vi "SMTP Email Get Literal Search Pattern.vi"(2 "case matching (sensitive)":T1=enum."system", 3 "literal string":string) -> (1 "regular expression":string)   [LabVIEW 2011, in "NewNI_SMTPEmail.lvlib"]
doc: "Builds a regular expression (used by Match Pattern) to match a literal string.\n\nWhen match case is FALSE, the regular expression will perform a case-insensitive match."
uses:
  NewNI_SMTPEmail.lvlib
  SMTP Email Case Matching.ctl
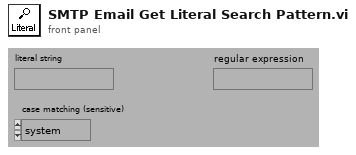
[diagram p1: front panel]
types:
  T1 = typedef "NewNI_SMTPEmail.lvlib/SMTP Email Case Matching.ctl" = enum16{"a != A", "a == A", "system"}
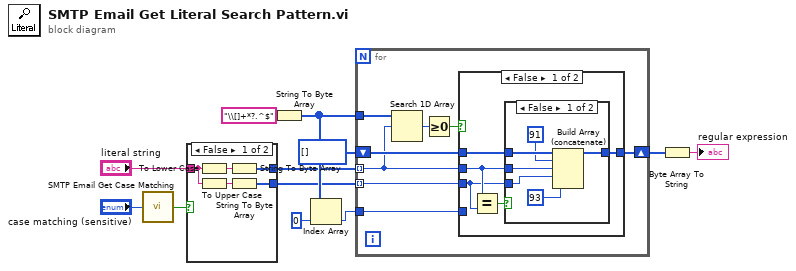
[diagram p0: block diagram]
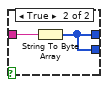
[diagram p2: hidden frame]
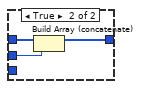
[diagram p3: hidden frame]
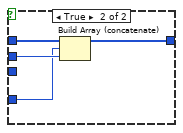
[diagram p4: hidden frame]
diagram:
  n1 = call "SMTP Email Get Case Matching.vi"("string matching"="case matching (sensitive)") -> ("match case"=w1:bool)
  n2 = case shown="False" w1 {
    tunnel: "literal string" -> [w14 w19]
    tunnel: [w17 w18] -> w4
    tunnel: [w13 w18] -> w3
    frame False {
      n3 = To Lower Case(string=w14) -> (all lower case string=w16:string)
      n4 = To Upper Case(1:w14) -> (0:w15:string)
      n5 = String To Byte Array(string=w16) -> (unsigned byte array=w17:u8[])
      n6 = String To Byte Array(string=w15) -> (unsigned byte array=w13:u8[])
    }
    frame True {
      n7 = String To Byte Array(string=w19) -> (unsigned byte array=w18:u8[])
    }
  }
  n8 = String To Byte Array(string="\\[]+*?.^$") -> (unsigned byte array=w11:u8[])
  n9 = Index Array(array=w11, index=0) -> (element=w9:u8)
  n10 = for {
    shift-right: [w22] -> w7
    shift-left: u8[] [] -> [w24]
    tunnel: w11 -> [w27]
    tunnel: w4 -> [w23] mode=indexing
    tunnel: w9 -> [w21]
    tunnel: w3 -> [w20] mode=indexing
    n11 = Search 1D Array(1D array=w27, element=w23) -> (index of element=w26:i32)  [unwired: 1 out]
    n12 = Greater Or Equal To 0?(x=w26) -> (x >= 0?=w25:bool)
    n13 = case shown="False" w25 {
      tunnel: w24 -> [w32 w45]
      tunnel: w23 -> [w30 w44]
      tunnel: [w31 w43] -> w22
      tunnel: w21 -> [_ w42]
      tunnel: w20 -> [w28 _]
      frame False {
        n14 = Equal?(x=w30, y=w28) -> (x = y?=w29:bool)
        n15 = case shown="False" w29 {
          tunnel: w30 -> [w36 w41]
          tunnel: [w38 w40] -> w31
          tunnel: w32 -> [w37 w39]
          tunnel: w28 -> [w35 _]
          frame False {
            n16 = Build Array (concatenate)(w37, u8 91, w36, w35, u8 93) -> (w38:u8[])
          }
          frame True {
            n17 = Build Array (concatenate)(w39, w41) -> (w40:u8[])
          }
        }
      }
      frame True {
        n18 = Build Array (concatenate)(w45, w42, w44) -> (w43:u8[])
      }
    }
  }
  n19 = Byte Array To String(unsigned byte array=w7) -> (string=→"regular expression":string)
